vi "Setter Generation tester.vi"() -> ()   [LabVIEW 2020, in "Method Generation.lvlib" / "Setter Generator.lvclass"]
uses:
  Setter Generator.lvclass
  Setter Generator.lvclass/Setter Generator.ctl
panel:
  out "error out":errorcluster
  out "Attributes":map{string, refnum<vi>}(c390)
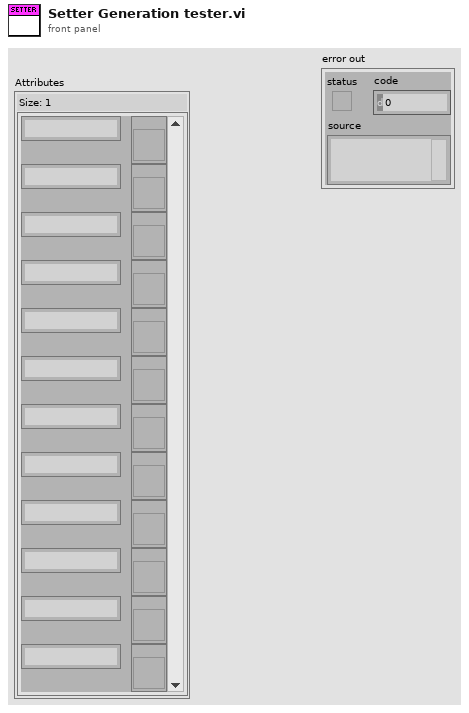
[diagram p1: front panel]
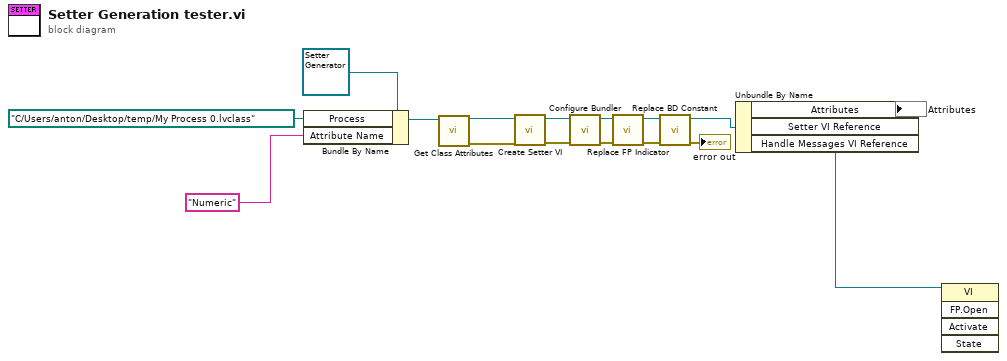
[diagram p0: block diagram]
diagram:
  n1 = Bundle By Name(cluster=refnum<class "Setter Generator.lvclass"> refnum ("New Getter Dialog In"), "Process"=path "C:/Users/anton/Desktop/temp/My Process 0.lvclass", "Attribute Name"="Numeric") -> (w15:refnum<class "Setter Generator.lvclass">)
  n2 = call "Get Class Attributes.vi"("Setter Generator In"=w15) -> ("error out"=w11:errorcluster, "Setter Generator Out"=w13:refnum<class "Setter Generator.lvclass">)  [unwired: 9 in]
  n3 = call "Create Setter VI.vi"("error in (no error)"=w11, "Setter Generator In"=w13) -> ("error out"=w9:errorcluster, "Setter Generator Out"=w12:refnum<class "Setter Generator.lvclass">)  [unwired: 8 in]
  n4 = call "Configure Bundler.vi"("error in (no error)"=w9, "Setter Generator In"=w12) -> ("error out"=w5:errorcluster, "Setter Generator Out"=w8:refnum<class "Setter Generator.lvclass">)  [unwired: 8 in]
  n5 = call "Replace FP Indicator.vi"("error in (no error)"=w5, "Setter Generator In"=w8) -> ("error out"=w4:errorcluster, "Setter Generator Out"=w7:refnum<class "Setter Generator.lvclass">)  [unwired: 8 in]
  n6 = call "Replace BD Constant.vi"("error in (no error)"=w4, "Setter Generator In"=w7) -> ("error out"=→"error out":errorcluster, "Setter Generator Out"=w6:refnum<class "Setter Generator.lvclass">)  [unwired: 8 in]
  n7 = Unbundle By Name(w6) -> ("Attributes"=→"Attributes":map{string, refnum<vi>}, "Handle Messages VI Reference"=w1:refnum<vi>)  [unwired: 1 out]
  n8 = invoke class="VI" method="FP.Open"(reference=w1) -> ()  [unwired: 4 in, 5 out]
